vi "Write Duty Cycle %.vi"(8 "error in":errorcluster, 10 "Duty Cycle":u8 format="%d %", 11 "IWrite Duty Cycle in":refnum<class "IWrite Duty Cycle.lvclass">) -> (0 "error out":errorcluster, 3 "IWrite Duty Cycle out":refnum<class "IWrite Duty Cycle.lvclass">)   [LabVIEW 2024, in "IWrite Duty Cycle.lvclass"]
uses:
  IWrite Duty Cycle.lvclass
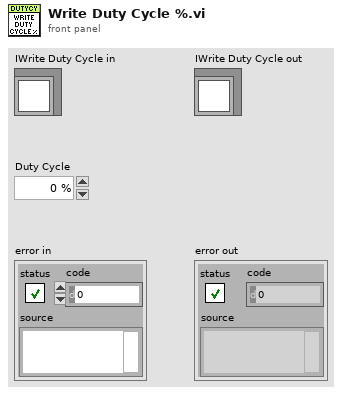
[diagram p1: front panel]
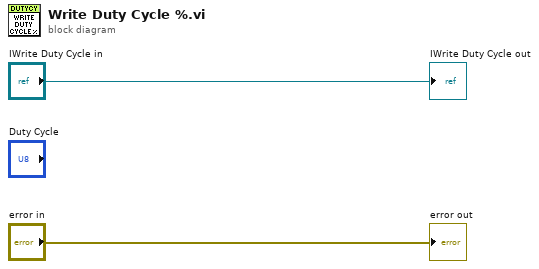
[diagram p0: block diagram]
diagram:
  "error out" <- "error in"
  "IWrite Duty Cycle out" <- "IWrite Duty Cycle in"
